vi "sg Set Multitone.vi"(6 "phase":u32(ring) items=["sgParabolic", "sgRandom", "sgRandomFixedSeed", "sgZeroPhase"], 7 "notchWidth":dbl, 8 "error in (no error)":errorcluster, 9 "spacing":dbl, 10 "count":i32, 11 "device":i32) -> (0 "error out":errorcluster, 3 "function return":u32(ring))   [LabVIEW 2014, in "VSG25A.lvlib"]
doc: "SG_API sgStatus sgSetMultitone(int device, int count, double spacing, double notchWidth, sgMultiTonePhase phase);"
uses:
  VSG25A.lvlib
  sg_api.dll
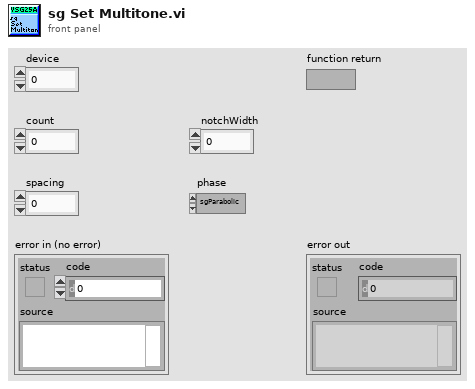
[diagram p1: front panel]
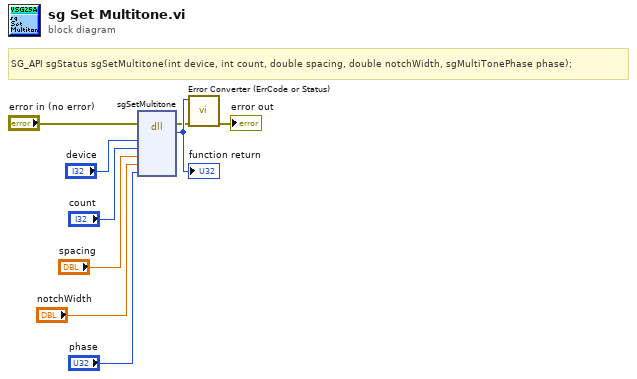
[diagram p0: block diagram]
diagram:
  # "SG_API sgStatus sgSetMultitone(int device, int count, double spacing, double notchWidth, sgMultiTonePhase phase);"
  n1 = dll-call lib="C:/Users/M_LAPTOP/Desktop/Labview/practice/VSG25A/sg_lib/sg_api.*" fn="sgSetMultitone"(error in="error in (no error)", "device"="device", "count"="count", "spacing"="spacing", "notchWidth"="notchWidth", "phase"="phase") -> (error out=w2:errorcluster, w9:u32)  [unwired: 7 in, 1 out]
  "function return" <- w9
  n2 = call "Error Converter (ErrCode or Status).vi"("error in (no error)"=w2, "error code"=w9) -> ("error out"=→"error out":errorcluster)  [unwired: 9 in]
